vi "4155C SampleI Config SMUs v2.0.vi"(4 "Sample I - Probe 4 (Disabled)":u32(ring)=3 items=["SMU1  ", "SMU2  ", "SMU3  ", "SMU4  ", "SMU5  ", "SMU6  "], 5 "Sample I - Drain/Gate":u32(ring)=1 items=["SMU1  ", "SMU2  ", "SMU3  ", "SMU4  ", "SMU5  ", "SMU6  "], 6 "Sample I - Probe 3 (Disabled)":u32(ring)=2 items=["SMU1  ", "SMU2  ", "SMU3  ", "SMU4  ", "SMU5  ", "SMU6  "], 7 "Sample I - Source/Common":u32(ring) items=["SMU1  ", "SMU2  ", "SMU3  ", "SMU4  ", "SMU5  ", "SMU6  "], 8 "error in (no error)":errorcluster, 9 "Gate Standby":bool, 10 "Drain Standby":bool, 11 "VISA resource name in":refnum<visa-resource-name>) -> (0 "error out":errorcluster, 3 "VISA Resource Name out":refnum<visa-resource-name>)   [LabVIEW 2016]
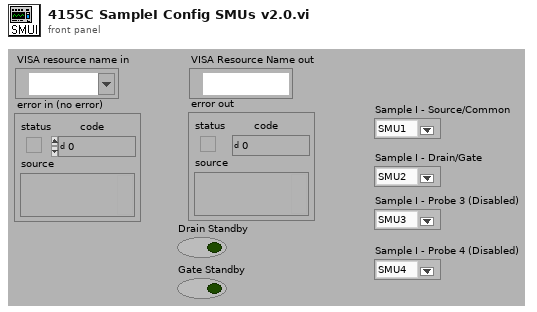
[diagram p1: front panel]
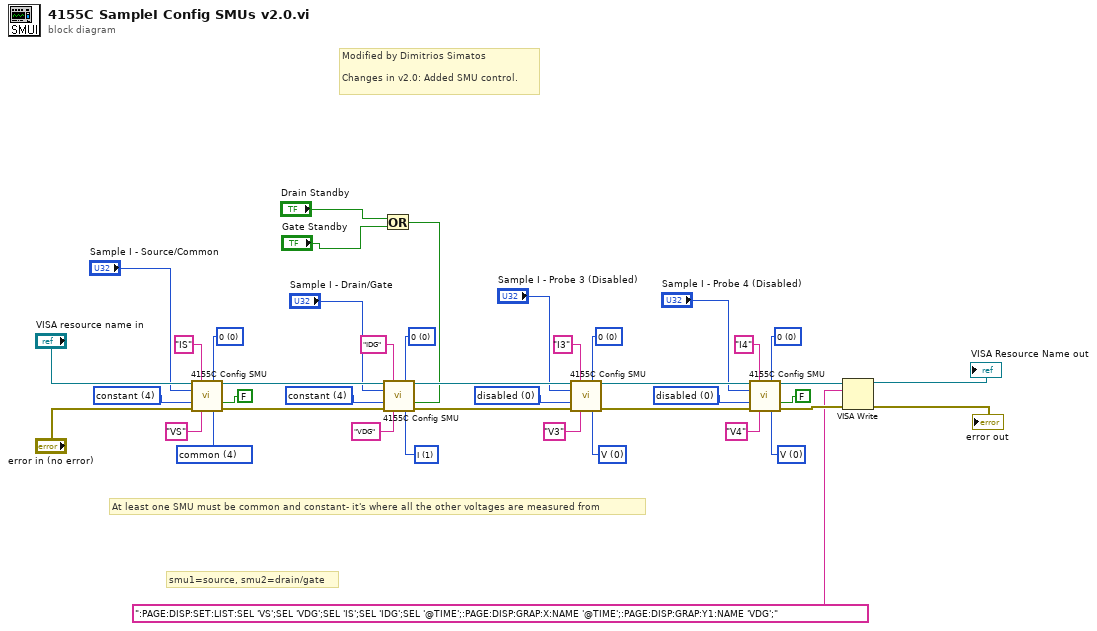
[diagram p0: block diagram]
diagram:
  w21 = u32 0 items=["V  ", "I  ", "V pulse  ", "I pulse  ", "  common  "] ("mode")
  w22 = u32 0 items=["0  ", "10K Ohms  ", "100K Ohms  ", "1M Ohms  "] ("series resistance *")
  w24 = u32 0 items=["disabled  ", "VAR1  ", "VAR2  ", "VAR1'  ", "constant  "] ("function")
  w26 = u32 0 items=["V  ", "I  ", "V pulse  ", "I pulse  ", "  common  "] ("mode")
  w27 = u32 0 items=["0  ", "10K Ohms  ", "100K Ohms  ", "1M Ohms  "] ("series resistance *")
  w29 = u32 0 items=["disabled  ", "VAR1  ", "VAR2  ", "VAR1'  ", "constant  "] ("function")
  w31 = u32 1 items=["V  ", "I  ", "V pulse  ", "I pulse  ", "  common  "] ("mode")
  w32 = u32 0 items=["0  ", "10K Ohms  ", "100K Ohms  ", "1M Ohms  "] ("series resistance *")
  w34 = u32 4 items=["disabled  ", "VAR1  ", "VAR2  ", "VAR1'  ", "constant  "] ("function")
  w37 = u32 4 items=["V  ", "I  ", "V pulse  ", "I pulse  ", "  common  "] ("mode")
  w38 = u32 0 items=["0  ", "10K Ohms  ", "100K Ohms  ", "1M Ohms  "] ("series resistance *")
  w40 = u32 4 items=["disabled  ", "VAR1  ", "VAR2  ", "VAR1'  ", "constant  "] ("function")
  # "Modified by Dimitrios Simatos\n\nChanges in v2.0: Added SMU control."
  # "smu1=source, smu2=drain/gate"
  # "At least one SMU must be common and constant- it's where all the other voltages are measured from"
  n1 = call "4155C Config SMU.vi"("VISA session"="VISA resource name in", "I name (max 6 chars)"="IS", "series resistance *"=w38, "unit to configure"="Sample I - Source/Common", "function"=w40, "standby"=FALSE, "error in (no error)"="error in (no error)", "V name (max 6 chars)"="VS", "mode"=w37) -> ("dup VISA resource name"=w18:refnum<visa-resource-name>, "error out"=w17:errorcluster)  [unwired: 5 in]
  n2 = Or(x="Drain Standby", y="Gate Standby") -> (x .or. y?=w5:bool)
  n3 = call "4155C Config SMU.vi"("VISA session"=w18, "I name (max 6 chars)"="IDG", "series resistance *"=w32, "unit to configure"="Sample I - Drain/Gate", "function"=w34, "standby"=w5, "error in (no error)"=w17, "V name (max 6 chars)"="VDG", "mode"=w31) -> ("dup VISA resource name"=w15:refnum<visa-resource-name>, "error out"=w16:errorcluster)  [unwired: 5 in]
  n4 = call "4155C Config SMU.vi"("VISA session"=w15, "I name (max 6 chars)"="I3", "series resistance *"=w27, "unit to configure"="Sample I - Probe 3 (Disabled)", "function"=w29, "error in (no error)"=w16, "V name (max 6 chars)"="V3", "mode"=w26) -> ("dup VISA resource name"=w14:refnum<visa-resource-name>, "error out"=w13:errorcluster)  [unwired: 6 in]
  n5 = call "4155C Config SMU.vi"("VISA session"=w14, "I name (max 6 chars)"="I4", "series resistance *"=w22, "unit to configure"="Sample I - Probe 4 (Disabled)", "function"=w24, "standby"=FALSE, "error in (no error)"=w13, "V name (max 6 chars)"="V4", "mode"=w21) -> ("dup VISA resource name"=w12:refnum<visa-resource-name>, "error out"=w11:errorcluster)  [unwired: 5 in]
  n6 = VISA Write(VISA resource name=w12, write buffer=":PAGE:DISP:SET:LIST:SEL 'VS';SEL 'VDG';SEL 'IS';SEL 'IDG';SEL '@TIME';:PAGE:DISP:GRAP:X:NAME '@TIME';:PAGE:DISP:GRAP:Y1:NAME 'VDG';" ("write buffer (\"\")"), error in (no error)=w11) -> (VISA resource name out=→"VISA Resource Name out":refnum<visa-resource-name>, error out=→"error out":errorcluster)  [unwired: 1 out]
